vi "simplePID Memory Write.vi"(0 "memory in":refnum<k21>="PID Data", 1 "channel (0)":u8, 2 "Input Selector":u8, 11 "state in":T1) -> ()   [LabVIEW 2020]
uses:
  <vilib>/rvi/Analysis/control/PID/Typedef/niFpgaPID_PIDMemoryItem.ctl
  <vilib>/rvi/DataTransferAndStorage/Container/XNode/niFpgaContainer.xnode
  <vilib>/rvi/Memory/Memory_Emulation/niFpgaMemoryEmulationRefIn.vi
  <vilib>/rvi/Analysis/control/PID/Typedef/niFpgaPID_PIDState.ctl
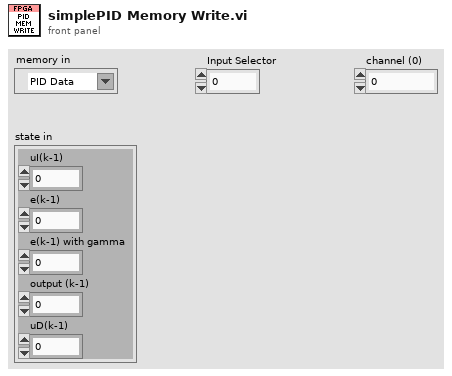
[diagram p1: front panel]
types:
  T1 = typedef "niFpgaPID_PIDState.ctl" = cluster{"uI(k-1)":sgl, "e(k-1)":sgl, "e(k-1) with gamma":sgl, "output (k-1)":sgl, "uD(k-1)":sgl}
  T2 = typedef "niFpgaPID_PIDMemoryItem.ctl" = cluster{"data 1":sgl, "data 2":sgl, "data 3":sgl, "data 4":sgl, "data 5":sgl}
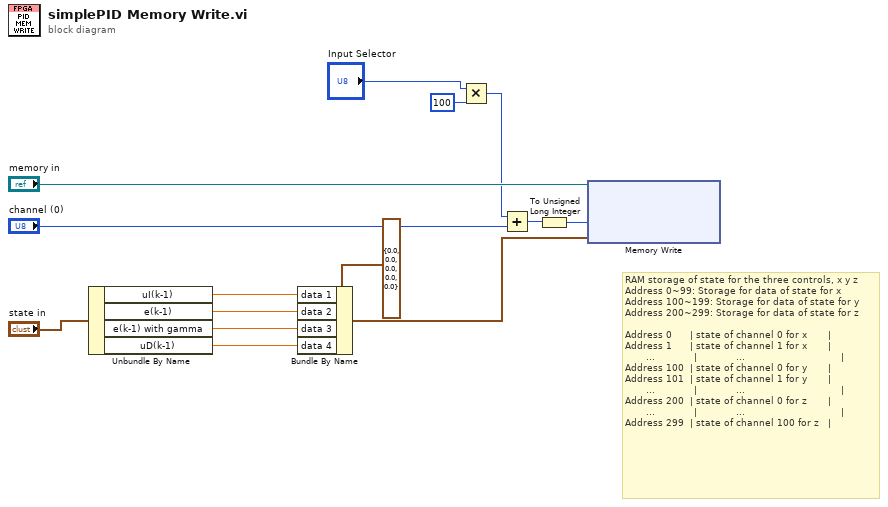
[diagram p0: block diagram]
diagram:
  # "RAM storage of state for the three controls, x y z\nAddress 0~99: Storage for data of state for x\nAddress 100~199: Storage for data of state for y\nAddress 200~299: Storage for data of state for z \n                                                                        \nAddress 0      | state of channel 0 for x       | \nAddress 1      | state of channel 1 for x       | \n       ...             |             ...                                |\nAddress 100  | state of channel 0 for y       | \nAddress 101  | state of channel 1 for y       | \n       ...             |             ...                                |\nAddress 200  | state of channel 0 for z       | \n       ...             |             ...                                |\nAddress 299  | state of channel 100 for z   |"
  n1 = Unbundle By Name("state in") -> ("uI(k-1)"=w13:sgl, "e(k-1)"=w10:sgl, "e(k-1) with gamma"=w11:sgl, "uD(k-1)"=w12:sgl)
  n2 = Bundle By Name(cluster=T2 {"data 1"=0.0, "data 2"=0.0, "data 3"=0.0, "data 4"=0.0, "data 5"=0.0} ("PID memory dummy type"), "data 1"=w13, "data 2"=w10, "data 3"=w11, "data 4"=w12) -> (w6:T2)
  n3 = Multiply(x="Input Selector", y=u8 100) -> (x*y=w2:u8)
  n4 = Add(x=w2, y="channel (0)") -> (x+y=w3:u8)
  n5 = To Unsigned Long Integer(number=w3) -> (unsigned 32bit integer=w9:u32)
  n6 = xnode ("Memory Write")("Address"=w9, "Data"=w6, "Memory In"="memory in") -> ()  [unwired: 1 out]
